vi "ROS_Topic_Init.vi"(0 "Definitions":T1={"Topic"="/robot/head/command_head_nod", "Type"="std_msgs/Bool", "Action"=enum."Publisher", "Update (ms)"=1, "queue size"=1}, 1 "node":string) -> (2 "ROS out":T3={"topic port"=0, "Node"="", "topic"="", "type"="", "node port"=0, "error "={"status"=FALSE, "code"=0, "source"=""}, "Direction"=enum."Node", "Update (ms)"=1, "FIFO size"=1}, 4 "error out":errorcluster)   [LabVIEW 2016]
doc: "Initializes a topic and returns a ROS cluster. Required before any read or write call."
uses:
  SubVIs/_ROSControl.ctl
  SubVIs/_ROSDirection.ctl
  Console/Servers/ServerSubs/TopicDef.ctl
  _ROSDefinition.vi
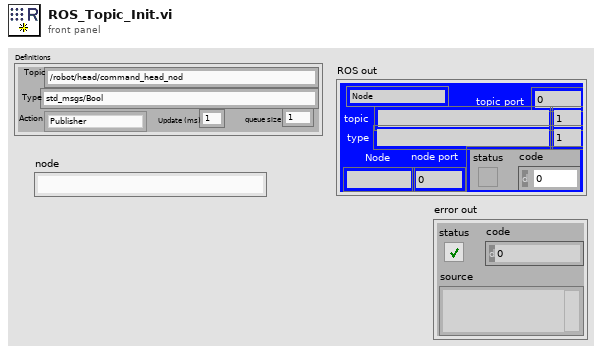
[diagram p1: front panel]
types:
  T1 = typedef "TopicDef.ctl" = cluster{"Topic":string, "Type":string, "Action":T2, "Update (ms)":u16, "queue size":u16}
  T2 = typedef "_ROSDirection.ctl" = enum16{"Node", "Publisher", "Subscriber", "ServiceClient", "ServiceProvider"}
  T3 = typedef "_ROSControl.ctl" = cluster{"topic port":u16, "Node":string, "topic":string, "type":string, "node port":u16, "error ":errorcluster, "Direction":T2, "Update (ms)":u16, "FIFO size":u16}
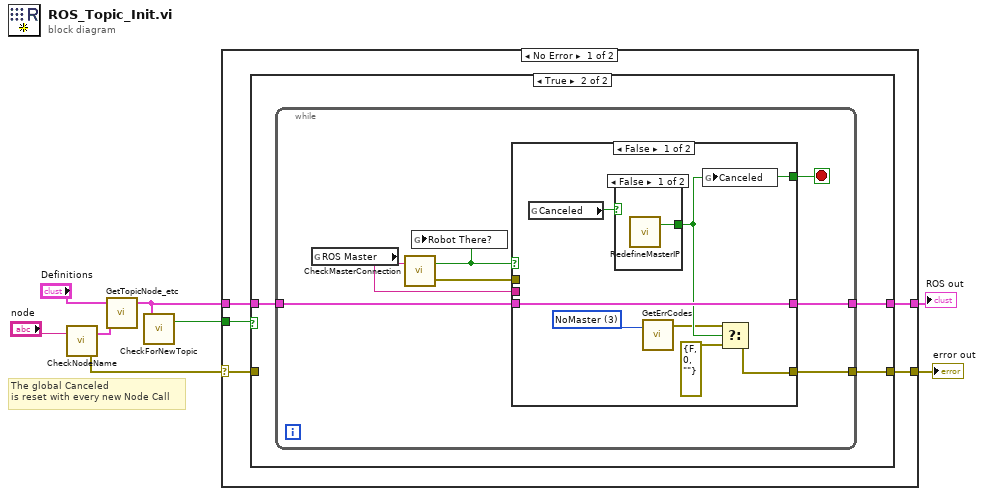
[diagram p0: block diagram]
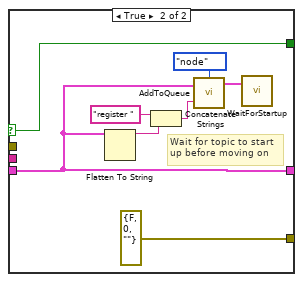
[diagram p4: hidden frame]
diagram:
  # "The global Canceled\nis reset with every new Node Call"
  n1 = call "CheckNodeName.vi"("node"="node") -> ("error out"=w1:errorcluster, "Node"=w6:cluster{"name":string, "Port":u16})  [unwired: 1 in]
  n2 = call "GetTopicNode_etc.vi"("Node"=w6, "Definitions"="Definitions") -> ("ROS"=w5:T3)  [unwired: 3 in]
  n3 = call "CheckForNewTopic.vi"("ROS"=w5) -> ("new?"=w4:bool)  [unwired: 2 in]
  n4 = case shown="No Error" w1 {
    selector: w1 -> [w9 w44]
    tunnel: [w13 w43] -> w7
    tunnel: w5 -> [w12 w43]
    tunnel: w4 -> [w11 _]
    tunnel: [w10 w44] -> w2
    frame No Error {
      n5 = case shown="True" w11 {
        tunnel: w12 -> [w15 w18]
        tunnel: [w15 w17] -> w13
        tunnel: [w14 w16] -> w10
        tunnel: w9 -> [w14 _]
        frame False {
        }
        frame True {
          n6 = while {
            tunnel: w18 -> [w25]
            tunnel: [w21] -> w17
            tunnel: [w19] -> w16
            stop <- w20 stop-if-true
            n7 = global read "_ROSDefinition.vi" "ROS Master"() -> (w24:string)
            n8 = call "CheckMasterConnection.vi"("Master IP"=w24) -> ("error out"=w23:errorcluster, "Master There?"=w22:bool)  [unwired: 1 in]
            n9 = global write "_ROSDefinition.vi" "Robot There?"(w22) -> ()
            n10 = case shown="False" w22 {
              selector: w22 -> [_ w40]
              tunnel: w25 -> [w31 w36]
              tunnel: [w31 w36] -> w21
              tunnel: w24 -> [_ _]
              tunnel: w23 -> [_ _]
              tunnel: [w29 w40] -> w20
              tunnel: [w32 errorcluster {"status"=FALSE, "code"=0, "source"=""} ("error out")] -> w19
              frame False {
                w30 = u16 3 items=["TopicReadTimeout", "Read=SS", "GetQueueErr", "NoMaster"] ("Error")
                n11 = global read "_ROSDefinition.vi" "Canceled"() -> (w28:bool)
                n12 = case shown="False" w28 {
                  selector: w28 -> [_ w34]
                  tunnel: [w33 w34] -> w29
                  frame False {
                    n13 = call "RedefineMasterIP.vi"() -> ("Abort?"=w33:bool)  [unwired: 2 in]
                  }
                  frame True {
                  }
                }
                n14 = call "GetErrCodes.vi"("Error"=w30) -> ("Error"=w27:errorcluster)  [unwired: 1 in]
                n15 = global write "_ROSDefinition.vi" "Canceled"(w29) -> ()
                n16 = Select(t=w27, s=w29, f=errorcluster {"status"=FALSE, "code"=0, "source"=""} ("error out")) -> (s? t:f=w32:errorcluster)
              }
              frame True {
                # "Wait for topic to start\nup before moving on"
                n17 = Flatten To String(anything=w36) -> (data string=w42:string)  [unwired: 3 in, 2 out]
                n18 = Concatenate Strings("register " ("string"), w42) -> (w37:string)
                n19 = call "AddToQueue.vi"("Cmd"=w37, "ROS"=w36, "Type"=enum16{"topic", "node"}."node" ("Name")) -> ("ROS out"=w35:T3)  [unwired: 2 in]
                n20 = call "WaitForStartup.vi"("ROS"=w35) -> ()  [unwired: 2 in, 1 out]
              }
            }
          }
        }
      }
    }
    frame Error {
    }
  }
  "ROS out" <- w7
  "error out" <- w2
